vi "Lakeshore 331 Test Program.vi"() -> ()   [LabVIEW 2022 SP3]
uses:
  <instrlib>/Lake Shore Cryotronics 331/Lake Shore Cryotronics 331.lvlib
panel:
  out "Setpoint":dbl min=-273.0 max=300000.0 step=0.0001 format="%.4f"
  out "error out":errorcluster
  in  "VISA resource name":refnum<visa-resource-name>
  out "Kelvin Reading":dbl min=0.0 max=1645.0 step=1e-05 format="%^.5e"
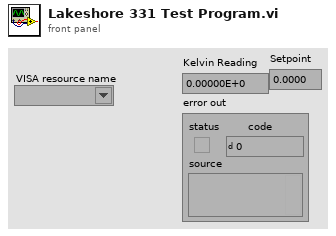
[diagram p1: front panel]
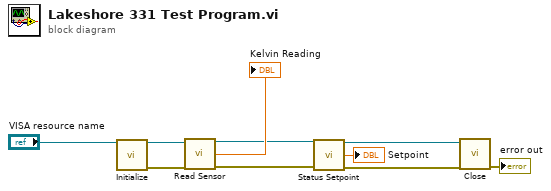
[diagram p0: block diagram]
diagram:
  n1 = call <instrlib>:"Initialize.vi"("VISA resource name"="VISA resource name") -> ("VISA resource name out"=w10:refnum<visa-resource-name>, "error out"=w8:errorcluster)  [unwired: 13 in]
  n2 = call <instrlib>:"Read Sensor.vi"("VISA resource name"=w10, "error in (no error)"=w8) -> ("VISA resource name out"=w5:refnum<visa-resource-name>, "Kelvin Reading"=→"Kelvin Reading":dbl, "error out"=w4:errorcluster)  [unwired: 9 in, 2 out]
  n3 = call <instrlib>:"Status Setpoint.vi"("VISA resource name"=w5, "error in (no error)"=w4) -> ("VISA resource name out"=w2:refnum<visa-resource-name>, "Setpoint"=→"Setpoint":dbl, "error out"=w3:errorcluster)  [unwired: 11 in]
  n4 = call <instrlib>:"Close.vi"("VISA resource name"=w2, "error in (no error)"=w3) -> ("error out"=→"error out":errorcluster)  [unwired: 13 in]
